vi "2_AdvancedDemo_MHHisto.vi"() -> ()   [LabVIEW 2010]
uses:
  Types/MH_UIThread_Cmds.ctl
  _lib/PQ/MultiHarp/MH_InitInfo.ctl
  Types/MH_UIThread_Data.ctl
  Types/MH_InputChannel.ctl
  _lib/PQ/MultiHarp/MH_RefSource.ctl
  _lib/PQ/MultiHarp/mhlib_x86_x64_UIThread.llb/MH_DllPath_global.vi
  <vilib>/Utility/error.llb/DialogType.ctl
  _lib/PQ/MultiHarp/MH_LibVersion_global.vi
  _lib/PQ/MultiHarp/MH_MeasMode.ctl
  Types/MH_SetInpChanData.ctl
  Types/MH_SetInpChanCmds.ctl
panel:
  in  "Settings":bool=TRUE
  in  "Run continuously":bool=TRUE caption="Conti."
  in  "Start":bool
  in  "Scale":bool
  out "CountRates":i32[](graph)
  in  "AllChannels":T1={"Enable"=TRUE, "Offset"=0, "Level"=-100, "Edge"=0, "DeadTime"=1000, "UseDeadTime"=FALSE, "SetEnableAllChan"=TRUE, "SetEdgeAllChan"=TRUE, "SetLevelAllChan"=TRUE, "SetOffsetAllChan"=TRUE, "SetUseDTAllChan"=TRUE, "SetDeadTAllChan"=TRUE} {"DeadTime" min=800 max=160000 step=1; "Edge" items=["falling", "rising"]; "Offset" min=-100000 max=100000 step=80; "Level" min=-1200 max=1200 step=1}
  in  "HistoLength":i32(ring)=6 caption="Num Bins" items=["1024", "2048", "4096", "8192", "16384", "32768", "65536"]
  in  "OvlLevel":u32=4294967295 caption="Ovl.Level" min=1 step=1
  in  "StopOvl.":bool=TRUE
  in  "AcqTime":i32=1000 caption="Acqu.           ms" min=1 max=360000 step=1
  in  "Binning":i32(ring) caption="Resol.            ps" items=["80", "160", "320", "640", "1280", "2560", "5120", "10240", "20480", "40960", "81920", "163840", "327680", "655360", "1310720", "2621440", "5242880", "10485760", "20971520", "41943040", "83886080", "167772160", "335544320"]
  in  "HistoOffset":i32 caption="Offset            ns" min=0 max=100000000 step=1
  out "HistoGraph":T2(graph)={0.0, "Resolution"=0.08, "Histogram"=[]}
  in  "SyncDeadTime":i32=1000 caption="Dead T.   ps" min=800 max=160000 step=1
  in  "UseDeadTime":bool caption="Use DT."
  in  "SyncEdge":i32(ring) caption="Edge" items=["falling", "rising"]
  in  "SyncDivider":i32(ring) caption="Divider" items=["1", "2", "4", "8", "16"]
  in  "SyncOffset":i32 caption="Offset      ps" min=-100000 max=100000 step=80
  in  "SyncLevel":i32=-100 caption="Level      mV" min=-1200 max=1200 step=1
  in  "Channels":T3[](array[typedef])=[{"Name"="Inp.Chan 1", "Enable"=TRUE, "Edge"=0, "Level"=-100, "Offset"=0, "UseDeadTime"=FALSE, "DeadTime"=1000}, {"Name"="Inp.Chan 2", "Enable"=TRUE, "Edge"=0, "Level"=-100, "Offset"=0, "UseDeadTime"=FALSE, "DeadTime"=1000}, {"Name"="Inp.Chan 3", "Enable"=TRUE, "Edge"=0, "Level"=-100, "Offset"=0, "UseDeadTime"=FALSE, "DeadTime"=1000}, {"Name"="Inp.Chan 4", "Enable"=TRUE, "Edge"=0, "Level"=-100, "Offset"=0, "UseDeadTime"=FALSE, "DeadTime"=1000}, {"Name"="Inp.Chan 5", "Enable"=TRUE, "Edge"=0, "Level"=-100, "Offset"=0, "UseDeadTime"=FALSE, "DeadTime"=1000}, {"Name"="Inp.Chan 6", "Enable"=TRUE, "Edge"=0, "Level"=-100, "Offset"=0, "UseDeadTime"=FALSE, "DeadTime"=1000}, {"Name"="Inp.Chan 7", "Enable"=TRUE, "Edge"=0, "Level"=-100, "Offset"=0, "UseDeadTime"=FALSE, "DeadTime"=1000}, {"Name"="Inp.Chan 8", "Enable"=TRUE, "Edge"=0, "Level"=-100, "Offset"=0, "UseDeadTime"=FALSE, "DeadTime"=1000}, {"Name"="Inp.Chan 9", "Enable"=TRUE, "Edge"=0, "Level"=-100, "Offset"=0, "UseDeadTime"=FALSE, "DeadTime"=1000}, {"Name"="Inp.Chan 10", "Enable"=TRUE, "Edge"=0, "Level"=-100, "Offset"=0, "UseDeadTime"=FALSE, "DeadTime"=1000}, {"Name"="Inp.Chan 11", "Enable"=TRUE, "Edge"=0, "Level"=-100, "Offset"=0, "UseDeadTime"=FALSE, "DeadTime"=1000}, {"Name"="Inp.Chan 12", "Enable"=TRUE, "Edge"=0, "Level"=-100, "Offset"=0, "UseDeadTime"=FALSE, "DeadTime"=1000}, {"Name"="Inp.Chan 13", "Enable"=TRUE, "Edge"=0, "Level"=-100, "Offset"=0, "UseDeadTime"=FALSE, "DeadTime"=1000}, {"Name"="Inp.Chan 14", "Enable"=TRUE, "Edge"=0, "Level"=-100, "Offset"=0, "UseDeadTime"=FALSE, "DeadTime"=1000}, {"Name"="Inp.Chan 15", "Enable"=TRUE, "Edge"=0, "Level"=-100, "Offset"=0, "UseDeadTime"=FALSE, "DeadTime"=1000}, {"Name"="Inp.Chan 16", "Enable"=TRUE, "Edge"=0, "Level"=-100, "Offset"=0, "UseDeadTime"=FALSE, "DeadTime"=1000}] {"DeadTime" min=800 max=160000 step=1; "Edge" items=["falling", "rising"]; "Offset" min=-100000 max=100000 step=80; "Level" min=-1200 max=1200 step=1}
  out "SyncRate":string="Sync Rate: 4999950 cps\n"
  out "OverFlow":bool caption="Overflow:"
  out "Status":string="Readout Rate: 8.6 Hz\t\tTotal Counts:\t\tCh. 1: 0 cnts.\t\tCh. 2: 1962112 cnts.\t\tCh. 3: 0 cnts.\t\tCh. 4: 1962112 cnts.\t\tCh. 5: 0 cnts.\t\tCh. 6: 1962112 cnts.\t\tCh. 7: 0 cnts.\t\tCh. 8: 1962112 cnts.\t\tCh. 9: 1962113 cnts.\t\tCh.10: 0 cnts.\t\tCh.11: 1962113 cnts.\t\tCh.12: 0 cnts.\t\tCh.13: 1962113 cnts.\t\tCh.14: 0 cnts.\t\tCh.15: 1962113 cnts.\t\tCh.16: 1962113 cnts.\t\t"
  # "Acquisition"
  # "All Channels"
  # "Sync"
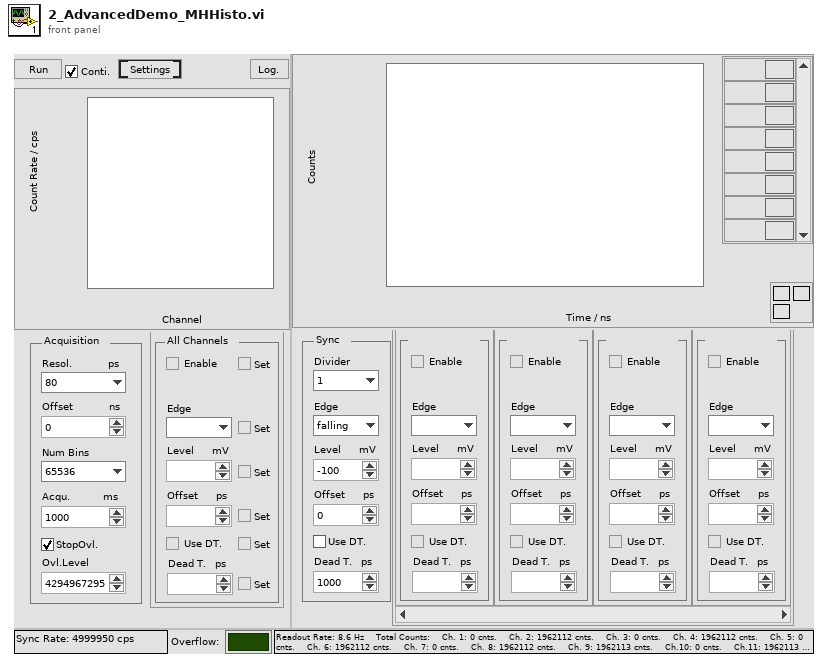
[diagram p1: front panel]
types:
  T1 = cluster{"Enable":bool, "Offset":i32, "Level":i32, "Edge":i32, "DeadTime":i32, "UseDeadTime":bool, "SetEnableAllChan":bool, "SetEdgeAllChan":bool, "SetLevelAllChan":bool, "SetOffsetAllChan":bool, "SetUseDTAllChan":bool, "SetDeadTAllChan":bool}
  T2 = cluster{dbl, "Resolution":dbl, "Histogram":u32[][]}
  T3 = typedef "MH_InputChannel.ctl" = cluster{"Name":string, "Enable":bool, "Edge":i32, "Level":i32, "Offset":i32, "UseDeadTime":bool, "DeadTime":i32}
  T4 = typedef "MH_UIThread_Data.ctl" = cluster{"Init Info":T5, "DevIdx":i32, "SyncDivider":i32, "SyncOffset":i32, "SyncLevel":i32, "Channels":T3[], "CurrentChannels":i32[], "AcqTime":i32, "Binning":i32, "HistoOffset":i32, "HistoLen":i32, "StopOvl.":bool, "OvlLevel":u32, "SyncEdge":i32, "StartMeas":bool, "HistoLength":i32, "Resolution":dbl, "Run cont.":bool, "Status":string, "SyncRate":i32, "BitShift":i32, "HistoAcqTime":dbl, "SyncRateStart":i32, "UseDeadTime":bool, "SyncDeadTime":i32, "SetInpChan":T6[]}
  T5 = typedef "MH_InitInfo.ctl" = cluster{"Library Version":string, "Serial No.":string, "Model":string, "Partnum":string, "Version":string, "features":i32, "nchannels":i32, "Base Resolution":dbl, "Bin Steps":i32}
  T6 = typedef "MH_SetInpChanData.ctl" = cluster{"Channel":i32, "Cmds":T7[], "Changed":cluster{"Name":bool, "Enable":bool, "Edge":bool, "Level":bool, "Offset":bool, "UseDeadTime":bool, "DeadTime":bool}}
  T7 = typedef "MH_SetInpChanCmds.ctl" = enum16{"SetInpChanEnable", "SetInpChanOffset", "SetInpChanDeadTime", "SetInpChanTrg"}
  T8 = typedef "MH_UIThread_Cmds.ctl" = enum16{"Idle", "Init", "SetInpChan", "SetSyncDivider", "SetSyncTrg", "SetSyncOffset", "SetSyncDeadTime", "SetBinning", "SetHistoOffset", "SetHistoLen", "SetStopOvl", "SetBitShift", "SetHistoAcqTime", "GetRates", "GetAllRates", "StartMeas", "StopMeas", "AbortMeas", "GetResolution", "GetHistos", "GetAllHistos", "ReadFiFo", "WriteStatus", "Resize", "EnableControls", "DisableControls", "Error", "Exit"}
  T9 = enum8{"Enabled", "Disabled", "Disabled and Grayed Out"}
  T10 = cluster{"[0]":bool, "[1]":bool, "[2]":bool, "[3]":bool, "[4]":bool, "[5]":bool}
  T11 = typedef "MH_MeasMode.ctl" = i32
  T12 = typedef "MH_RefSource.ctl" = enum16{"INTERNAL", "EXTERNAL_10MHZ", "WR_MASTER_GENERIC", "WR_SLAVE_GENERIC", "WR_GRANDM_GENERIC", "EXTN_GPS_PPS", "EXTN_GPS_PPS_UART", "WR_MASTER_MHARP", "WR_SLAVE_MHARP", "WR_GRANDM_MHARP"}
  T13 = cluster{dbl, "Resolution":dbl, "Histograms":u32[][]}
  T14 = typedef "DialogType.ctl" = u16
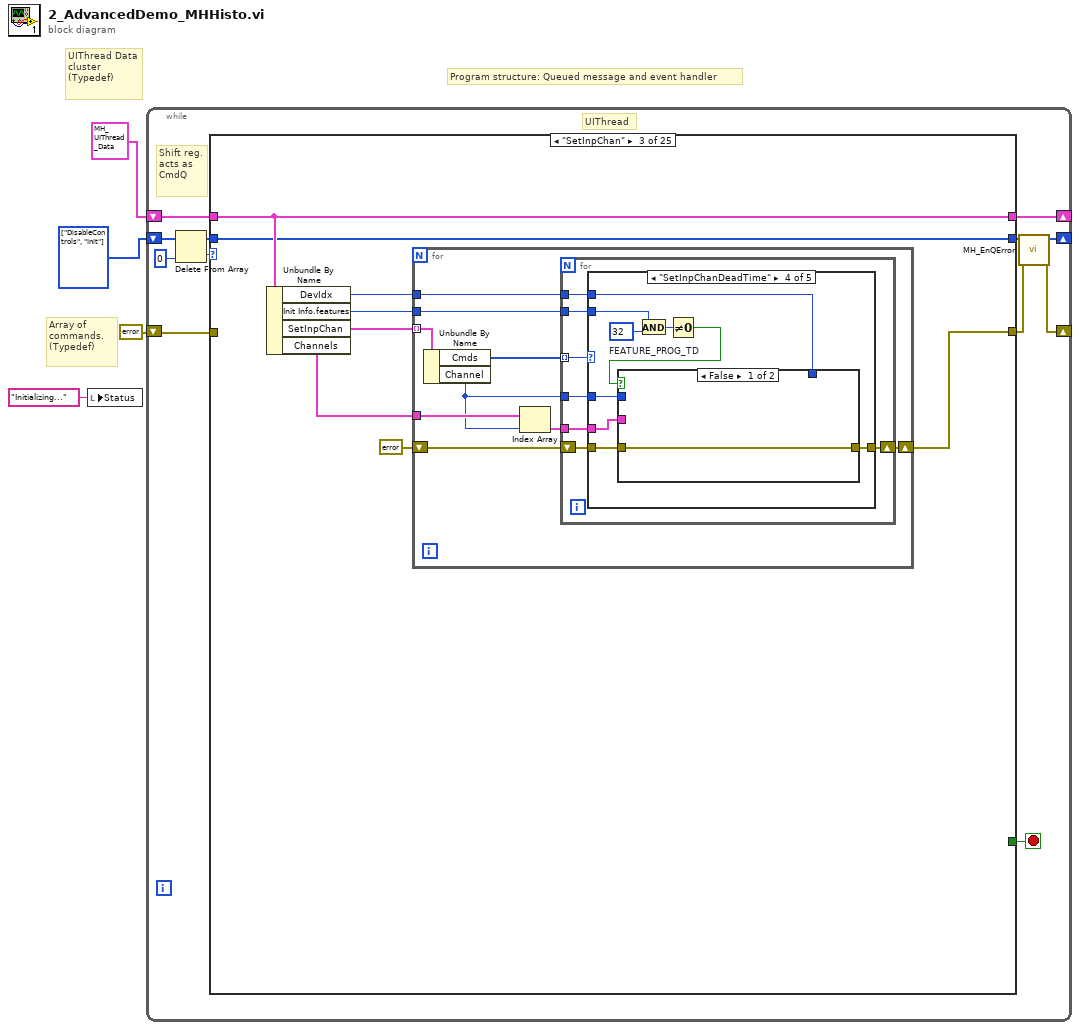
[diagram p0: block diagram]
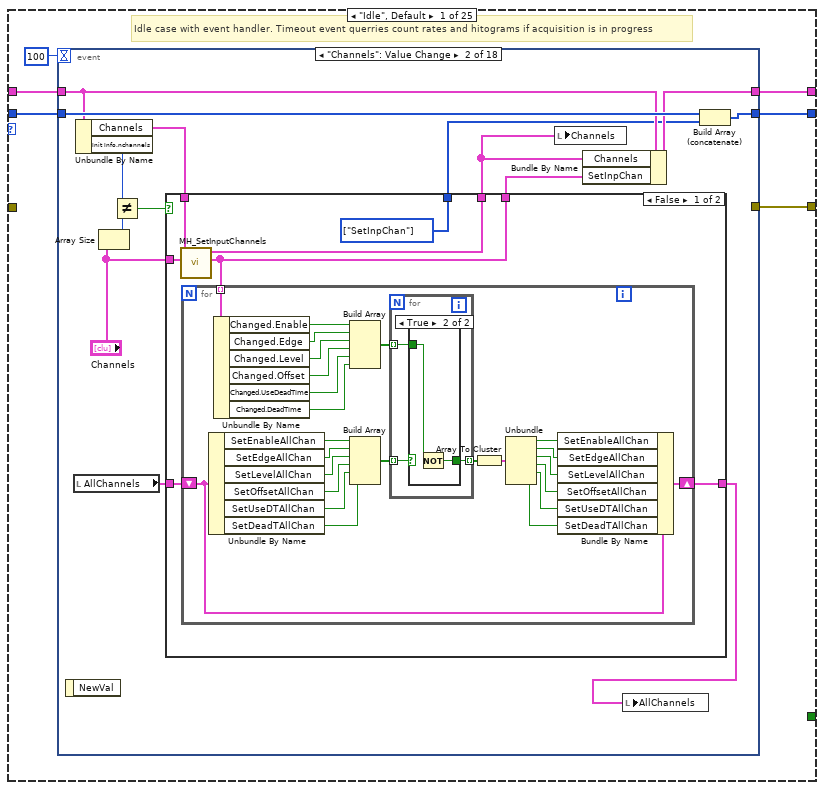
[diagram p2: hidden frame]
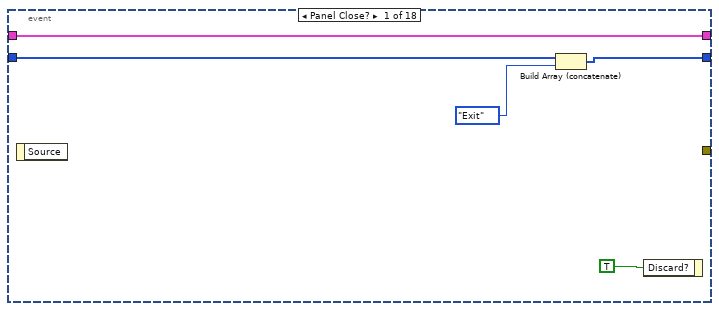
[diagram p3: hidden frame]
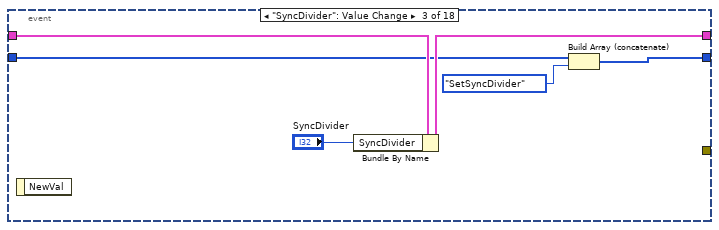
[diagram p6: hidden frame]
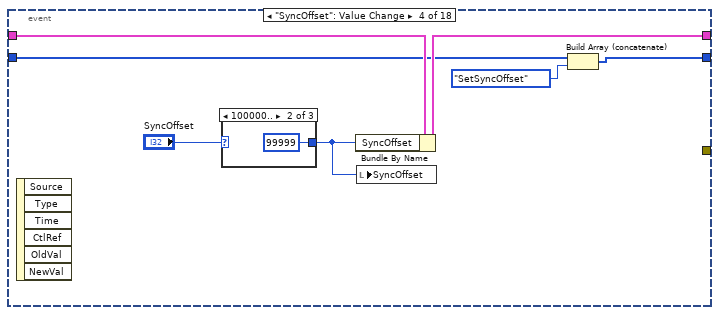
[diagram p7: hidden frame]
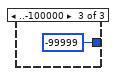
[diagram p9: hidden frame]
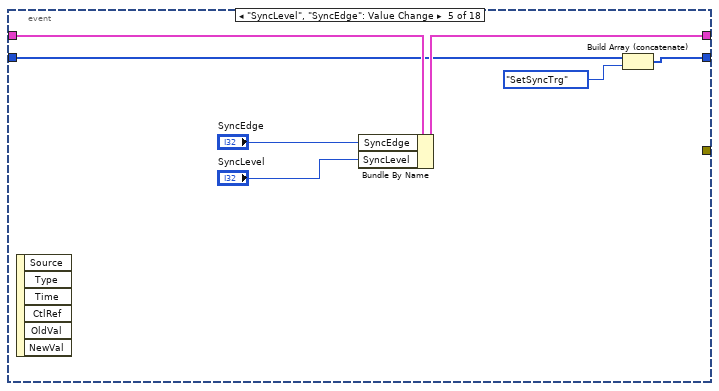
[diagram p10: hidden frame]
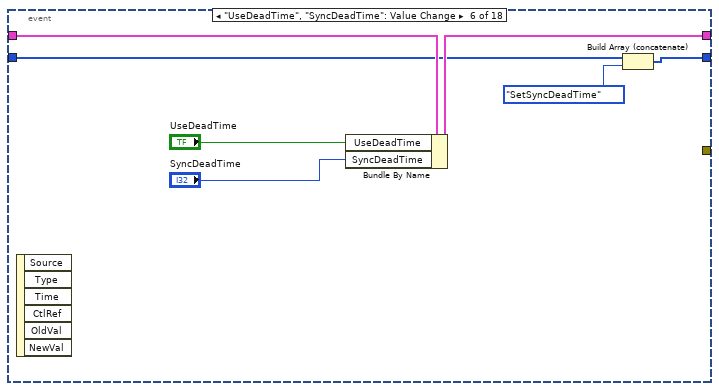
[diagram p11: hidden frame]
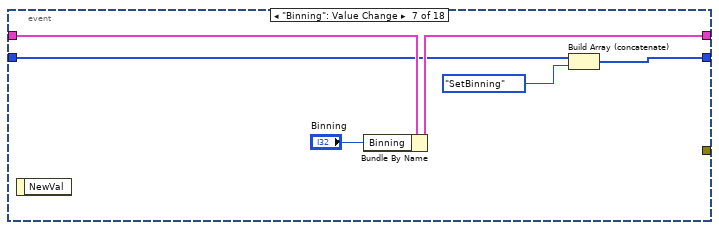
[diagram p12: hidden frame]
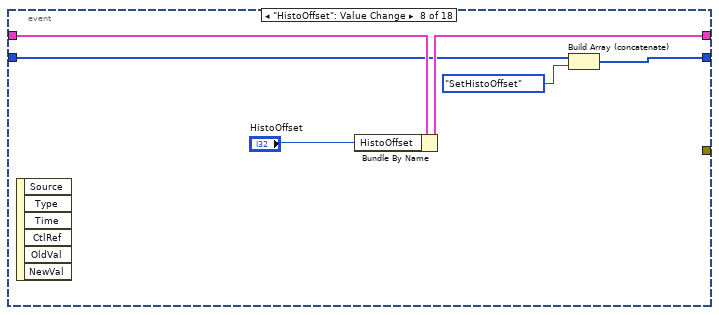
[diagram p13: hidden frame]
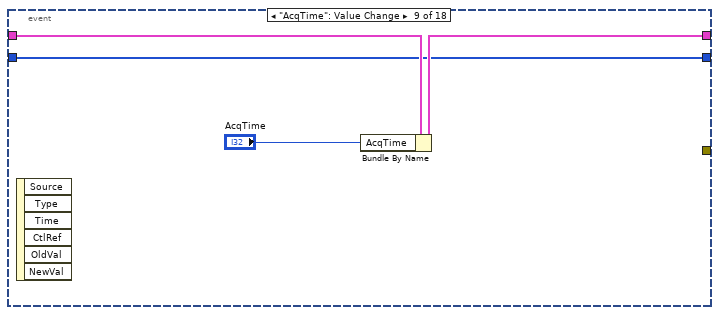
[diagram p14: hidden frame]
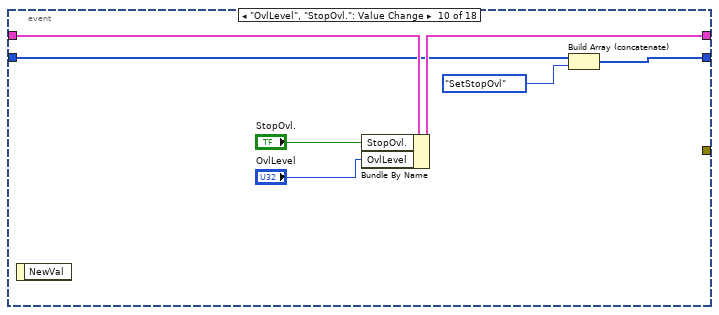
[diagram p15: hidden frame]
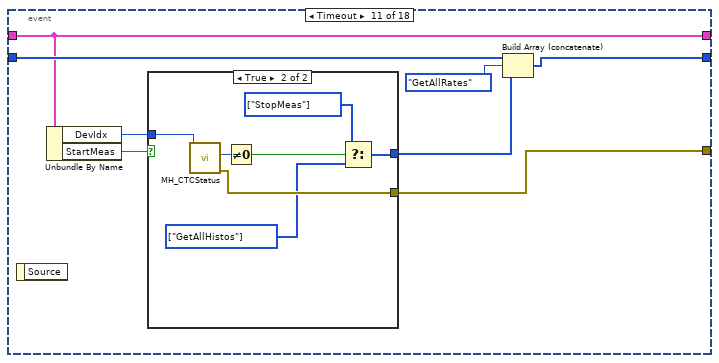
[diagram p16: hidden frame]
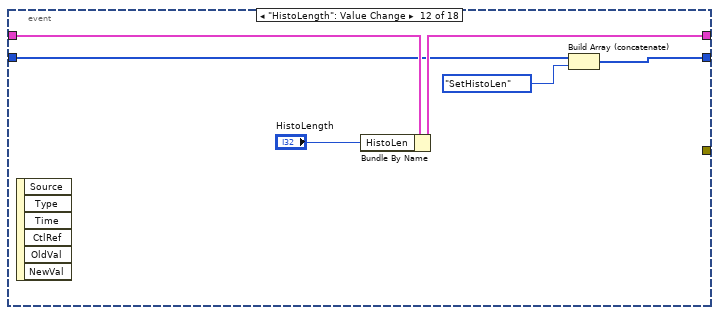
[diagram p18: hidden frame]
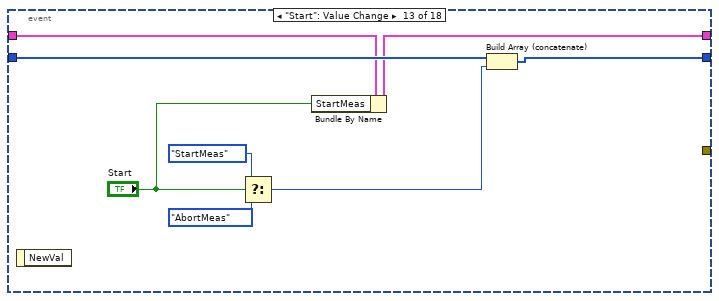
[diagram p19: hidden frame]
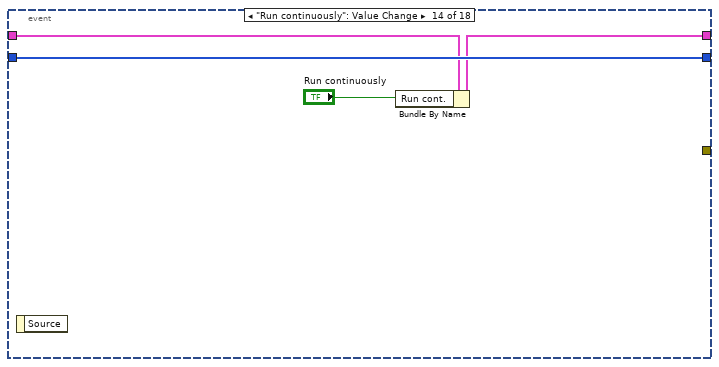
[diagram p20: hidden frame]
diagram:
  w3 = T8[] [enum."DisableControls", enum."Init"] items=["Idle", "Init", "SetInpChan", "SetSyncDivider", "SetSyncTrg", "SetSyncOffset", "SetSyncDeadTime", "SetBinning", "SetHistoOffset", "SetHistoLen", "SetStopOvl", "SetBitShift", "SetHistoAcqTime", "GetRates", "GetAllRates", "StartMeas", "StopMeas", "AbortMeas", "GetResolution", "GetHistos", "GetAllHistos", "ReadFiFo", "WriteStatus", "Resize", "EnableControls", "DisableControls", "Error", "Exit"]
  # "Array of commands.\n(Typedef)"
  # "Program structure: Queued message and event handler"
  # "UIThread Data cluster\n(Typedef)"
  n1 = local write "Status"("Initializing..." ("Status")) -> ()
  n2 = while {
    shift-right: [w5] -> _
    shift-left: w3 -> [w12]
    shift-right: [w15] -> _
    shift-left: T4 {"Init Info"={"Library Version"="", "Serial No."="", "Model"="", "Partnum"="", "Version"="", "features"=0, "nchannels"=0, "Base Resolution"=0.0, "Bin Steps"=0}, "DevIdx"=0, "SyncDivider"=1, "SyncOffset"=0, "SyncLevel"=50, "Channels"=[], "CurrentChannels"=[], "AcqTime"=1, "Binning"=1, "HistoOffset"=1, "HistoLen"=1024, "StopOvl."=FALSE, "OvlLevel"=1024, "SyncEdge"=10, "StartMeas"=FALSE, "HistoLength"=0, "Resolution"=0.0, "Run cont."=FALSE, "Status"="", "SyncRate"=0, "BitShift"=0, "HistoAcqTime"=0.0, "SyncRateStart"=0, "UseDeadTime"=FALSE, "SyncDeadTime"=800, "SetInpChan"=[]} -> [w14]
    shift-right: [w7] -> _
    shift-left: errorcluster {"status"=FALSE, "code"=0, "source"=""} ("error IO") -> [w13]
    stop <- w16 stop-if-true
    # "Shift reg.\nacts as\nCmdQ"
    # "UIThread"
    n3 = Delete From Array(array=w12, index=0) -> (deleted portion=w10:T8, array with subset deleted=w9:T8[])  [unwired: 1 in]
    n4 = case shown="\"SetInpChan\"" w10 {
      tunnel: [w22 w304 w323 w385 w394 w406 w412 w419 w427 w435 w440 w451 w462 w477 w485 w499 w513 w538 w570 w594 w607 w614 w626 w632 w636] -> w6
      tunnel: [_ _ _ _ _ _ _ _ _ _ _ _ _ _ _ _ _ _ _ _ _ _ _ _ TRUE] -> w16
      tunnel: [w21 w284 w324 w387 w395 w407 w416 w423 w428 w430 w441 w450 w461 w483 w488 w502 w509 w537 w569 w593 w595 w613 w625 w633 w639] -> w15
      tunnel: w14 -> [w20 w289 w324 w387 w395 w407 w416 w423 w428 w431 w441 w450 w461 w483 w489 w503 w510 w537 w569 w593 w595 w613 w625 w633 w639]
      tunnel: [w17 w307 w321 w383 w393 w405 w415 w422 w426 w434 w439 w444 w460 w482 w491 w505 w511 w535 w565 _ _ _ _ _ w637] -> w8
      tunnel: w13 -> [_ _ _ _ _ _ _ _ _ _ _ _ _ _ _ _ _ _ _ _ _ _ _ w634 _]
      tunnel: w9 -> [w19 w306 w323 w385 w394 w406 w412 w418 w427 w435 w440 w451 w462 w478 w486 w500 w513 w538 w570 w594 w607 w614 w626 _ w636]
      frame "Idle", Default {
        # "Idle case with event handler. Timeout event querries count rates and hitograms if acquisition is in progress"
        n5 = event shown="[1] \"Channels\": Value Change" {
          selector: _ -> [_ _ _ _ _ _ _ _ _ _ _ _ _ _ _ _ _ _]
          dyn-events: _ -> [_ _ _ _ _ _ _ _ _ _ _ _ _ _ _ _ _ _]
          timeout: 100 -> [_ _ _ _ _ _ _ _ _ _ _ _ _ _ _ _ _ _]
          tunnel: [w23 w40 w82 w90 w99 w107 w113 w119 w124 w130 w140 w151 w159 w167 w173 w181 w191 w204] -> w22
          tunnel: [w26 w33 w86 w93 w103 w110 w116 w122 w126 w133 w139 w154 w157 w165 w172 w180 w194 w198] -> w21
          tunnel: w20 -> [w26 w35 w87 w94 w104 w111 w117 w123 w127 w134 w139 w155 w158 w166 w172 w180 w194 w199]
          tunnel: w19 -> [w25 w41 w84 w92 w101 w109 w115 w121 w124 w132 w142 w153 w161 w167 w173 w181 w192 w205]
          tunnel: [_ _ _ _ _ _ _ _ _ _ w135 _ _ _ _ _ _ _] -> w17
          event Panel Close? {
            n6 = event-data() -> ()  [unwired: 1 in, 1 out]
            n7 = Build Array (concatenate)(w25, MH_UIThread_Cmds."Exit") -> (w23:T8[])
            n8 = event-data("Discard?"=TRUE) -> ()  [unwired: 1 in, 1 out]
          }
          event "Channels": Value Change {
            n9 = event-data() -> ()  [unwired: 1 in, 1 out]
            n10 = local read "AllChannels"() -> (w29:T1)
            n11 = Unbundle By Name(w35) -> ("Channels"=w36:T3[], "Init Info.nchannels"=w39:i32)
            n12 = Array Size(array="Channels") -> (size(s)=w38:i32)
            n13 = Not Equal?(x=w39, y=w38) -> (x != y?=w37:bool)
            n14 = case shown="False" w37 {
              tunnel: "Channels" -> [w47 _]
              tunnel: [w46 w81] -> w34
              tunnel: w36 -> [w48 w81]
              tunnel: [w44 _] -> w32
              tunnel: [w45 _] -> w30
              tunnel: w29 -> [w43 w80]
              tunnel: [w42 w80] -> w28
              frame False {
                w45 = T8[] [enum."SetInpChan"] items=["Idle", "Init", "SetInpChan", "SetSyncDivider", "SetSyncTrg", "SetSyncOffset", "SetSyncDeadTime", "SetBinning", "SetHistoOffset", "SetHistoLen", "SetStopOvl", "SetBitShift", "SetHistoAcqTime", "GetRates", "GetAllRates", "StartMeas", "StopMeas", "AbortMeas", "GetResolution", "GetHistos", "GetAllHistos", "ReadFiFo", "WriteStatus", "Resize", "EnableControls", "DisableControls", "Error", "Exit"] ("array")
                n15 = call "MH_SetInputChannels.vi"("Channels new"=w47, "Channels old"=w48) -> ("SetInpChan"=w44:T6[], "Channels"=w46:T3[])  [unwired: 8 in]
                n16 = for {
                  tunnel: w44 -> [w73] mode=indexing
                  shift-right: [w55] -> w42
                  shift-left: w43 -> [w57]
                  n17 = Unbundle By Name(w57) -> ("SetEnableAllChan"=w66:bool, "SetEdgeAllChan"=w65:bool, "SetLevelAllChan"=w64:bool, "SetOffsetAllChan"=w63:bool, "SetUseDTAllChan"=w62:bool, "SetDeadTAllChan"=w61:bool)
                  n18 = Unbundle By Name(w73) -> ("Changed.Enable"=w72:bool, "Changed.Edge"=w71:bool, "Changed.Level"=w70:bool, "Changed.Offset"=w69:bool, "Changed.UseDeadTime"=w68:bool, "Changed.DeadTime"=w67:bool)
                  n19 = Build Array(w72, w71, w70, w69, w68, w67) -> (w59:bool[])
                  n20 = Build Array(w66, w65, w64, w63, w62, w61) -> (w60:bool[])
                  n21 = for {
                    tunnel: w60 -> [w76] mode=indexing
                    tunnel: w59 -> [w74] mode=indexing
                    tunnel: [w75] -> w58 mode=indexing
                    n22 = case shown="True" w76 {
                      selector: w76 -> [w77 _]
                      tunnel: [w77 w78] -> w75
                      tunnel: w74 -> [_ w79]
                      frame False {
                      }
                      frame True {
                        n23 = Not(x=w79) -> (.not. x?=w78:bool)
                      }
                    }
                  }
                  n24 = Array To Cluster(array=w58) -> (cluster=w56:T10)
                  n25 = Unbundle(w56) -> ("[0]"=w54:bool, "[1]"=w53:bool, "[2]"=w52:bool, "[3]"=w51:bool, "[4]"=w50:bool, "[5]"=w49:bool)
                  n26 = Bundle By Name(cluster=w57, "SetEnableAllChan"=w54, "SetEdgeAllChan"=w53, "SetLevelAllChan"=w52, "SetOffsetAllChan"=w51, "SetUseDTAllChan"=w50, "SetDeadTAllChan"=w49) -> (w55:T1)
                }
              }
              frame True {
              }
            }
            n27 = local write "Channels"(w34) -> ()
            n28 = Bundle By Name(cluster=w35, "Channels"=w34, "SetInpChan"=w32) -> (w33:T4)
            n29 = local write "AllChannels"(w28) -> ()
            n30 = Build Array (concatenate)(w41, w30) -> (w40:T8[])
          }
          event "SyncDivider": Value Change {
            n31 = event-data() -> ()  [unwired: 1 in, 1 out]
            n32 = Bundle By Name(cluster=w87, "SyncDivider"="SyncDivider") -> (w86:T4)
            n33 = Build Array (concatenate)(w84, MH_UIThread_Cmds."SetSyncDivider") -> (w82:T8[])
          }
          event "SyncOffset": Value Change {
            n34 = event-data() -> ()  [unwired: 1 in, 6 out]
            n35 = case shown="100000.." "SyncOffset" {
              selector: "SyncOffset" -> [w95 _ _]
              tunnel: [w95 99999 ("SyncOffset") -99999 ("SyncOffset")] -> w88
              frame Default {
              }
              frame 100000.. {
              }
              frame ..-100000 {
              }
            }
            n36 = Bundle By Name(cluster=w94, "SyncOffset"=w88) -> (w93:T4)
            n37 = local write "SyncOffset"(w88) -> ()
            n38 = Build Array (concatenate)(w92, MH_UIThread_Cmds."SetSyncOffset") -> (w90:T8[])
          }
          event "SyncLevel", "SyncEdge": Value Change {
            n39 = event-data() -> ()  [unwired: 1 in, 6 out]
            n40 = Bundle By Name(cluster=w104, "SyncEdge"="SyncEdge", "SyncLevel"="SyncLevel") -> (w103:T4)
            n41 = Build Array (concatenate)(w101, MH_UIThread_Cmds."SetSyncTrg") -> (w99:T8[])
          }
          event "UseDeadTime", "SyncDeadTime": Value Change {
            n42 = event-data() -> ()  [unwired: 1 in, 6 out]
            n43 = Bundle By Name(cluster=w111, "UseDeadTime"="UseDeadTime", "SyncDeadTime"="SyncDeadTime") -> (w110:T4)
            n44 = Build Array (concatenate)(w109, MH_UIThread_Cmds."SetSyncDeadTime") -> (w107:T8[])
          }
          event "Binning": Value Change {
            n45 = event-data() -> ()  [unwired: 1 in, 1 out]
            n46 = Bundle By Name(cluster=w117, "Binning"="Binning") -> (w116:T4)
            n47 = Build Array (concatenate)(w115, MH_UIThread_Cmds."SetBinning") -> (w113:T8[])
          }
          event "HistoOffset": Value Change {
            n48 = event-data() -> ()  [unwired: 1 in, 6 out]
            n49 = Bundle By Name(cluster=w123, "HistoOffset"="HistoOffset") -> (w122:T4)
            n50 = Build Array (concatenate)(w121, MH_UIThread_Cmds."SetHistoOffset") -> (w119:T8[])
          }
          event "AcqTime": Value Change {
            n51 = event-data() -> ()  [unwired: 1 in, 6 out]
            n52 = Bundle By Name(cluster=w127, "AcqTime"="AcqTime") -> (w126:T4)
          }
          event "OvlLevel", "StopOvl.": Value Change {
            n53 = event-data() -> ()  [unwired: 1 in, 1 out]
            n54 = Bundle By Name(cluster=w134, "StopOvl."="StopOvl.", "OvlLevel"="OvlLevel") -> (w133:T4)
            n55 = Build Array (concatenate)(w132, MH_UIThread_Cmds."SetStopOvl") -> (w130:T8[])
          }
          event Timeout {
            n56 = event-data() -> ()  [unwired: 1 in, 1 out]
            n57 = Unbundle By Name(w139) -> ("DevIdx"=w137:i32, "StartMeas"=w138:bool)
            n58 = case shown="True" w138 {
              tunnel: w137 -> [_ w149]
              tunnel: [_ w147] -> w136
              tunnel: [_ w145] -> w135
              frame False {
              }
              frame True {
                w143 = T8[] [enum."GetAllHistos"] items=["Idle", "Init", "SetInpChan", "SetSyncDivider", "SetSyncTrg", "SetSyncOffset", "SetSyncDeadTime", "SetBinning", "SetHistoOffset", "SetHistoLen", "SetStopOvl", "SetBitShift", "SetHistoAcqTime", "GetRates", "GetAllRates", "StartMeas", "StopMeas", "AbortMeas", "GetResolution", "GetHistos", "GetAllHistos", "ReadFiFo", "WriteStatus", "Resize", "EnableControls", "DisableControls", "Error", "Exit"]
                w146 = T8[] [enum."StopMeas"] items=["Idle", "Init", "SetInpChan", "SetSyncDivider", "SetSyncTrg", "SetSyncOffset", "SetSyncDeadTime", "SetBinning", "SetHistoOffset", "SetHistoLen", "SetStopOvl", "SetBitShift", "SetHistoAcqTime", "GetRates", "GetAllRates", "StartMeas", "StopMeas", "AbortMeas", "GetResolution", "GetHistos", "GetAllHistos", "ReadFiFo", "WriteStatus", "Resize", "EnableControls", "DisableControls", "Error", "Exit"]
                n59 = call "MH_CTCStatus.vi"("devidx"=w149) -> ("error out"=w145:errorcluster, "ctcstatus"=w148:i32)  [unwired: 8 in, 1 out]
                n60 = Not Equal To 0?(x=w148) -> (x != 0?=w144:bool)
                n61 = Select(t=w146, s=w144, f=w143) -> (s? t:f=w147:T8[])
              }
            }
            n62 = Build Array (concatenate)(w142, MH_UIThread_Cmds."GetAllRates", w136) -> (w140:T8[])
          }
          event "HistoLength": Value Change {
            n63 = event-data() -> ()  [unwired: 1 in, 6 out]
            n64 = Bundle By Name(cluster=w155, "HistoLen"="HistoLength") -> (w154:T4)
            n65 = Build Array (concatenate)(w153, MH_UIThread_Cmds."SetHistoLen") -> (w151:T8[])
          }
          event "Start": Value Change {
            n66 = event-data() -> ()  [unwired: 1 in, 1 out]
            n67 = Select(t=MH_UIThread_Cmds."StartMeas", s="Start", f=MH_UIThread_Cmds."AbortMeas") -> (s? t:f=w160:T8)
            n68 = Bundle By Name(cluster=w158, "StartMeas"="Start") -> (w157:T4)
            n69 = Build Array (concatenate)(w161, w160) -> (w159:T8[])
          }
          event "Run continuously": Value Change {
            n70 = event-data() -> ()  [unwired: 1 in, 1 out]
            n71 = Bundle By Name(cluster=w166, "Run cont."="Run continuously") -> (w165:T4)
          }
          event "Scale": Value Change {
            n72 = event-data() -> ()  [unwired: 1 in, 1 out]
            n73 = Select(t=u8 0 ("Y Scale.Mapping Mode"), s="Scale", f=u8 1 ("Y Scale.Mapping Mode")) -> (s? t:f=w168:u8)
            n74 = property on="HistoGraph" class="WFGraph (strict)"("YScale.Mapping Mode"=w168) -> ()  [unwired: 2 in, 2 out]
          }
          event "Settings": Value Change {
            n75 = event-data() -> ()  [unwired: 1 in, 1 out]
            n76 = property on="Splitter" class="Splitter"() -> ("Position"=w179:i32)  [unwired: 2 in, 2 out]
            n77 = Select(t=300 ("PosT"), s="Settings", f=0 ("PosF")) -> (s? t:f=w176:i32)
            n78 = Subtract(x=w179, y=w176) -> (x-y=w175:i32)
            n79 = while {
              shift-right: [w190] -> _
              shift-left: w175 -> [w183]
              i -> [w189]
              stop <- w186 stop-if-true
              n80 = property on="Splitter 4" class="Splitter"("Position"=w183) -> (error out=w182:errorcluster)  [unwired: 2 in, 1 out]
              n81 = Greater Or Equal?(x=w189, y=10) -> (x >= y?=w187:bool)
              n82 = Decrement(x=w183) -> (x-1=w190:i32)
              n83 = Unbundle(w182) -> ("status"=w185:bool)  [unwired: 2 out]
              n84 = Not(x=w185) -> (.not. x?=w184:bool)
              n85 = Or(x=w184, y=w187) -> (x .or. y?=w186:bool)
            }
          }
          event Panel Resize {
            n86 = event-data() -> ()  [unwired: 1 in, 1 out]
            n87 = Build Array (concatenate)(w192, MH_UIThread_Cmds."Resize") -> (w191:T8[])
          }
          event "AllChannels": Value Change {
            w196 = T8[] [enum."SetInpChan"] items=["Idle", "Init", "SetInpChan", "SetSyncDivider", "SetSyncTrg", "SetSyncOffset", "SetSyncDeadTime", "SetBinning", "SetHistoOffset", "SetHistoLen", "SetStopOvl", "SetBitShift", "SetHistoAcqTime", "GetRates", "GetAllRates", "StartMeas", "StopMeas", "AbortMeas", "GetResolution", "GetHistos", "GetAllHistos", "ReadFiFo", "WriteStatus", "Resize", "EnableControls", "DisableControls", "Error", "Exit"] ("array")
            n88 = event-data() -> ()  [unwired: 1 in, 1 out]
            n89 = local read "Channels"() -> (w203:T3[])
            n90 = for {
              tunnel: w203 -> [w208] mode=indexing
              tunnel: "AllChannels" -> [w207]
              tunnel: [w206] -> w201 mode=indexing
              n91 = Unbundle By Name(w207) -> ("SetEnableAllChan"=w209:bool, "SetEdgeAllChan"=w210:bool, "SetLevelAllChan"=w211:bool, "SetOffsetAllChan"=w212:bool, "SetUseDTAllChan"=w213:bool, "SetDeadTAllChan"=w214:bool)
              n92 = Build Array(w209, w210, w211, w212, w213, w214) -> (w215:bool[])
              n93 = for {
                tunnel: w215 -> [w220] mode=indexing
                shift-right: [w217] -> w206
                shift-left: w208 -> [w218]
                tunnel: w207 -> [w216]
                i -> [w219]
                n94 = case shown="True" w220 {
                  tunnel: w219 -> [_ w225]
                  tunnel: w216 -> [_ w224]
                  tunnel: w218 -> [w221 w223]
                  tunnel: [w221 w222] -> w217
                  frame False {
                  }
                  frame True {
                    n95 = case shown="Default" w225 {
                      tunnel: w224 -> [w229 w233 w237 w242 w249 w253 _]
                      tunnel: w223 -> [w228 w232 w236 w241 w248 w252 w254]
                      tunnel: [w226 w230 w234 w240 w246 w250 w254] -> w222
                      frame 0 {
                        n96 = Unbundle By Name(w229) -> ("Enable"=w227:bool)
                        n97 = Bundle By Name(cluster=w228, "Enable"=w227) -> (w226:T3)
                      }
                      frame 1 {
                        n98 = Unbundle By Name(w233) -> ("Edge"=w231:i32)
                        n99 = Bundle By Name(cluster=w232, "Edge"=w231) -> (w230:T3)
                      }
                      frame 2 {
                        n100 = Unbundle By Name(w237) -> ("Level"=w235:i32)
                        n101 = Bundle By Name(cluster=w236, "Level"=w235) -> (w234:T3)
                      }
                      frame 3 {
                        n102 = Unbundle By Name(w242) -> ("Offset"=w239:i32)
                        n103 = case shown="100000.." w239 {
                          selector: w239 -> [w243 _ _]
                          tunnel: [w243 99999 ("SyncOffset") -99999 ("SyncOffset")] -> w238
                          frame Default {
                          }
                          frame 100000.. {
                          }
                          frame ..-100000 {
                          }
                        }
                        n104 = Bundle By Name(cluster=w241, "Offset"=w238) -> (w240:T3)
                      }
                      frame 4 {
                        n105 = Unbundle By Name(w249) -> ("UseDeadTime"=w247:bool)
                        n106 = Bundle By Name(cluster=w248, "UseDeadTime"=w247) -> (w246:T3)
                      }
                      frame 5 {
                        n107 = Unbundle By Name(w253) -> ("DeadTime"=w251:i32)
                        n108 = Bundle By Name(cluster=w252, "DeadTime"=w251) -> (w250:T3)
                      }
                      frame Default {
                      }
                    }
                  }
                }
              }
            }
            n109 = Build Array (concatenate)(w205, w196) -> (w204:T8[])
            n110 = Unbundle By Name(w199) -> ("Channels"=w200:T3[])
            n111 = call "MH_SetInputChannels.vi"("Channels new"=w201, "Channels old"=w200) -> ("SetInpChan"=w197:T6[], "Channels"=w195:T3[])  [unwired: 8 in]
            n112 = local write "Channels"(w195) -> ()
            n113 = Bundle By Name(cluster=w199, "Channels"=w195, "SetInpChan"=w197) -> (w198:T4)
          }
        }
      }
      frame "Init" {
        w264 = 1000 ("SyncDeadTime")
        w265 = FALSE ("UseDeadTime")
        w267 = T11 0 items=["HIST"=0, "T2"=2, "T3"=3]  # Mode
        w277 = MH_RefSource."INTERNAL"  # refsource
        w291 = TRUE ("Run cont.")
        w293 = FALSE ("StartMeas")
        w294 = u32 4294967295 ("OvlLevel")
        w295 = TRUE ("StopOvl.")
        w296 = 6 ("HistoLen")
        w297 = 1000 ("AcqTime")
        w298 = 0 ("HistoOffset")
        w299 = 0 ("Binning")
        w300 = -100 ("SyncLevel")
        w301 = 0 ("SyncZeroX")
        w302 = 0 ("SyncOffset")
        w303 = 0 ("SyncDivider")
        w305 = T8[] [enum."SetSyncDivider", enum."SetSyncOffset", enum."SetSyncTrg", enum."SetSyncDeadTime", enum."SetInpChan", enum."SetBinning", enum."SetHistoOffset", enum."SetHistoLen", enum."SetStopOvl", enum."Resize", enum."EnableControls", enum."WriteStatus"] items=["Idle", "Init", "SetInpChan", "SetSyncDivider", "SetSyncTrg", "SetSyncOffset", "SetSyncDeadTime", "SetBinning", "SetHistoOffset", "SetHistoLen", "SetStopOvl", "SetBitShift", "SetHistoAcqTime", "GetRates", "GetAllRates", "StartMeas", "StopMeas", "AbortMeas", "GetResolution", "GetHistos", "GetAllHistos", "ReadFiFo", "WriteStatus", "Resize", "EnableControls", "DisableControls", "Error", "Exit"]
        # "Init HW"
        # "Set path to mhlib.dll"
        # "Init all FP controls and corresponding copy in UIThread Data cluster"
        # "EnQ list of commands"
        # "Array with Inp.Chan."
        # "Initialization: 1. Init HW -> get # of channels -> make array for Inp.Channels\n2. Init all FP controls and corresponding fields in UIThread Data cluster\n3. EnQ list of commands for further initialization"
        n114 = disable-structure shown="TARGET_TYPE==Windows, Default" {
          disable-tunnel: ["MHLib64" ("name or relative path") "MHLib" ("name or relative path")] -> w266
          frame condition #0 (active) {
          }
          frame condition #1 {
          }
        }
        n115 = call <vilib>:"Error Cluster From Error Code.vi"("is warning? (False)"=FALSE, "show call chain? (False)"=TRUE, "error message (\"\")"="DLL not found!" ("error message (\"\")"), "error code (0)"=5000) -> ("error out"=w278:errorcluster)  [unwired: 5 in]
        n116 = call "GetDLLPath.vi"("DllName_32bit"="MHLib" ("name or relative path"), "DllName_64bit"=w266) -> ("file exists?"=w280:bool, "DLLPath"=w281:path)  [unwired: 8 in]
        n117 = global write "MH_DllPath_global.vi" "DllPath"(w281) -> ()
        n118 = Build Array (concatenate)(w306, w305) -> (w304:T8[])
        n119 = Select(t=errorcluster {"status"=FALSE, "code"=0, "source"=""} ("error IO"), s=w280, f=w278) -> (s? t:f=w285:errorcluster)
        n120 = property on="AllChannels" class="Clust (strict)"("Val(Sgnl)"=T1 {"Enable"=TRUE, "Offset"=0, "Level"=-100, "Edge"=0, "DeadTime"=1000, "UseDeadTime"=FALSE, "SetEnableAllChan"=TRUE, "SetEdgeAllChan"=TRUE, "SetLevelAllChan"=TRUE, "SetOffsetAllChan"=TRUE, "SetUseDTAllChan"=TRUE, "SetDeadTAllChan"=TRUE} ("AllChannels")) -> ()  [unwired: 2 in, 2 out]
        n121 = property on="HistoGraph" class="WFGraph (strict)"("LegPlotMin"=u32 8 ("Legend:Plot Minimum")) -> ()  [unwired: 2 in, 2 out]
        n122 = property on="Settings" class="Bool (strict)"("Val(Sgnl)"=TRUE ("Value (Signaling)")) -> ()  [unwired: 2 in, 2 out]
        n123 = global read "MH_LibVersion_global.vi" "Library Version"() -> (w276:string)
        n124 = property on="Scale" class="Bool (strict)"("Val(Sgnl)"=FALSE ("Value (Signaling)")) -> ()  [unwired: 2 in, 2 out]
        n125 = call "InitMH_UIThread.vi"("error in (no error)"=w285, "Mode"=w267, "refsource"=w277, "Library Version"=w276) -> ("error out"=w307:errorcluster, "Init Info"=w309:T5, "DevIdx"=w308:i32)  [unwired: 5 in]
        n126 = local write "SyncDivider"(w303) -> ()
        n127 = local write "SyncOffset"(w302) -> ()
        n128 = local write "SyncEdge"(w301) -> ()
        n129 = local write "SyncLevel"(w300) -> ()
        n130 = local write "UseDeadTime"(w265) -> ()
        n131 = local write "SyncDeadTime"(w264) -> ()
        n132 = local write "Binning"(w299) -> ()
        n133 = local write "HistoOffset"(w298) -> ()
        n134 = local write "AcqTime"(w297) -> ()
        n135 = local write "HistoLength"(w296) -> ()
        n136 = local write "StopOvl."(w295) -> ()
        n137 = local write "OvlLevel"(w294) -> ()
        n138 = local write "Start"(w293) -> ()
        n139 = local write "Run continuously"(w291) -> ()
        n140 = Bundle By Name(cluster=w289, "DevIdx"=w308, "Init Info"=w309, "Status"="Initialized!") -> (w288:T4)
        n141 = Unbundle By Name(w288) -> ("Init Info.Bin Steps"=w287:i32, "Init Info.Base Resolution"=w270:dbl, "Init Info.nchannels"=w262:i32)
        n142 = Initialize Array(u32 0, w262, 1024 ("dimension size")) -> (w269:u32[][])
        n143 = call "MH_InitChannels.vi"("nchannels"=w262) -> ("SetInpChan"=w260:T6[], "Channels"=w261:T3[])  [unwired: 9 in]
        n144 = Divide(x=w270, y=1000.0) -> (x/y=w271:dbl)
        n145 = call "MH_CalcBinningValues.vi"("Bin Steps"=w287) -> ("BinningValues"=w292:cluster{"String":string, "Value":i32}[])  [unwired: 10 in]
        n146 = Bundle(0.0, w271, w269) -> (w263:cluster{dbl, dbl, u32[][]})  [unwired: 1 in]
        n147 = for {
          N: w262 -> [_]
          tunnel: w263 -> [w312]
          i -> [w314]
          n148 = Increment(x=w314) -> (x+1=w313:i32)
          n149 = Format Into String(format string="Ch.%d", w313) -> (resulting string=w315:string)  [unwired: 2 in, 1 out]
          n150 = property on="HistoGraph" class="WFGraph (strict)"("Value"=w312, "Active Plot"=w314, "Plot.Plot Name"=w315) -> ()  [unwired: 2 in, 2 out]
        }
        n151 = property on="Binning" class="Ring (strict)"("StringsAndValues[]"=w292) -> ()  [unwired: 2 in, 2 out]
        n152 = local write "Channels"(w261) -> ()
        n153 = Bundle By Name(cluster=w288, "Channels"=w261, "SetInpChan"=w260, "SyncDivider"=w303, "SyncOffset"=w302, "SyncEdge"=w301, "SyncLevel"=w300, "UseDeadTime"=w265, "SyncDeadTime"=w264, "Binning"=w299, "HistoOffset"=w298, "AcqTime"=w297, "HistoLen"=w296, "StopOvl."=w295, "OvlLevel"=w294, "StartMeas"=w293, "Run cont."=w291) -> (w284:T4)
      }
      frame "SetInpChan" {
        n154 = Unbundle By Name(w324) -> ("DevIdx"=w319:i32, "Init Info.features"=w317:i32, "SetInpChan"=w322:T6[], "Channels"=w318:T3[])
        n155 = for {
          tunnel: w318 -> [w329]
          tunnel: w322 -> [w333] mode=indexing
          shift-right: [w331] -> w321
          shift-left: errorcluster {"status"=FALSE, "code"=0, "source"=""} ("error out") -> [w330]
          tunnel: w319 -> [w327]
          tunnel: w317 -> [w325]
          n156 = Unbundle By Name(w333) -> ("Cmds"=w332:T7[], "Channel"=w326:i32)
          n157 = Index Array(array=w329, index=w326) -> (element=w328:T3)
          n158 = for {
            tunnel: w332 -> [w340] mode=indexing
            tunnel: w326 -> [w339]
            shift-right: [w338] -> w331
            shift-left: w330 -> [w337]
            tunnel: w328 -> [w336]
            tunnel: w327 -> [w335]
            tunnel: w325 -> [w334]
            n159 = case shown="\"SetInpChanDeadTime\"" w340 {
              tunnel: w339 -> [_ w346 w353 w358 w374]
              tunnel: [w341 w345 w352 w362 w379] -> w338
              tunnel: w337 -> [w341 w344 w351 w361 w378]
              tunnel: w336 -> [_ w343 w350 w360 w377]
              tunnel: w335 -> [_ w342 w349 w359 w376]
              tunnel: w334 -> [_ _ _ w355 _]
              frame Default {
              }
              frame "SetInpChanEnable" {
                n160 = Unbundle By Name(w343) -> ("Enable"=w347:bool)
                n161 = call "MH_SetInputChannelEnable.vi"("error in (no error)"=w344, "enable"=w347, "channel"=w346, "devidx"=w342) -> ("error out"=w345:errorcluster)  [unwired: 6 in, 1 out]
              }
              frame "SetInpChanOffset" {
                n162 = Unbundle By Name(w350) -> ("Offset"=w348:i32)
                n163 = call "MH_SetInputChannelOffset.vi"("error in (no error)"=w351, "Offset"=w348, "channel"=w353, "devidx"=w349) -> ("error out"=w352:errorcluster)  [unwired: 6 in, 1 out]
              }
              frame "SetInpChanDeadTime" {
                w356 = 32  # FEATURE_PROG_TD
                n164 = And(x=w355, y=w356) -> (x .and. y?=w357:i32)
                n165 = Not Equal To 0?(x=w357) -> (x != 0?=w354:bool)
                n166 = case shown="False" w354 {
                  tunnel: [w363 w372] -> w362
                  tunnel: w361 -> [w363 w371]
                  tunnel: w360 -> [_ w370]
                  tunnel: w359 -> [_ w369]
                  tunnel: w358 -> [_ w367]
                  frame False {
                  }
                  frame True {
                    n167 = Unbundle By Name(w370) -> ("UseDeadTime"=w366:bool, "DeadTime"=w368:i32)
                    n168 = Boolean To (0,1)(Boolean=w366) -> (0, 1=w365:i16)
                    n169 = To Long Integer(number=w365) -> (32bit integer=w364:i32)
                    n170 = call "MH_SetInputDeadTime.vi"("channel"=w367, "error in (no error)"=w371, "deadtime"=w368, "on"=w364, "devidx"=w369) -> ("error out"=w372:errorcluster)  [unwired: 5 in, 1 out]
                  }
                }
              }
              frame "SetInpChanTrg" {
                n171 = Unbundle By Name(w377) -> ("Level"=w373:i32, "Edge"=w375:i32)
                n172 = call "MH_SetInputEdgeTrg.vi"("channel"=w374, "error in (no error)"=w378, "edge"=w375, "level"=w373, "devidx"=w376) -> ("error out"=w379:errorcluster)  [unwired: 5 in, 1 out]
              }
            }
          }
        }
      }
      frame "SetSyncDivider" {
        n173 = Unbundle By Name(w387) -> ("DevIdx"=w386:i32, "SyncDivider"=w382:i32)
        n174 = Power Of 2(x=w382) -> (2^x=w381:dbl)
        n175 = To Long Integer(number=w381) -> (32bit integer=w380:i32)
        n176 = call "MH_SetSyncDiv.vi"("SyncDivider"=w380, "devidx"=w386) -> ("error out"=w384:errorcluster)  [unwired: 8 in, 1 out]
        n177 = flat-sequence {
          tunnel: w384 -> [w388]
          tunnel: [w388] -> w383
          frame #0 {
            n178 = Wait (ms)(milliseconds to wait=u32 100) -> ()  [unwired: 1 out]
          }
        }
      }
      frame "SetSyncTrg" {
        n179 = Unbundle By Name(w395) -> ("DevIdx"=w392:i32, "SyncLevel"=w390:i32, "SyncEdge"=w391:i32)
        n180 = call "MH_SetSyncEdgeTrg.vi"("edge"=w391, "level"=w390, "devidx"=w392) -> ("error out"=w393:errorcluster)  [unwired: 7 in, 1 out]
      }
      frame "SetSyncDeadTime" {
        w398 = 32  # FEATURE_PROG_TD
        n181 = Unbundle By Name(w407) -> ("DevIdx"=w404:i32, "UseDeadTime"=w402:bool, "SyncDeadTime"=w403:i32, "Init Info.features"=w397:i32)
        n182 = Boolean To (0,1)(Boolean=w402) -> (0, 1=w401:i16)
        n183 = And(x=w397, y=w398) -> (x .and. y?=w399:i32)
        n184 = To Long Integer(number=w401) -> (32bit integer=w400:i32)
        n185 = Not Equal To 0?(x=w399) -> (x != 0?=w396:bool)
        n186 = case shown="False" w396 {
          tunnel: [_ w411] -> w405
          tunnel: w404 -> [_ w410]
          tunnel: w403 -> [_ w409]
          tunnel: w400 -> [_ w408]
          frame False {
          }
          frame True {
            n187 = call "MH_SetSyncDeadTime.vi"("deadtime"=w409, "on"=w408, "devidx"=w410) -> ("error out"=w411:errorcluster)  [unwired: 7 in, 1 out]
          }
        }
      }
      frame "SetSyncOffset" {
        n188 = Unbundle By Name(w416) -> ("DevIdx"=w414:i32, "SyncOffset"=w413:i32)
        n189 = call "MH_SetSyncChannelOffset.vi"("Offset"=w413, "devidx"=w414) -> ("error out"=w415:errorcluster)  [unwired: 8 in, 1 out]
      }
      frame "SetBinning" {
        # "When binning is changed the new resolution is querried"
        n190 = Unbundle By Name(w423) -> ("DevIdx"=w421:i32, "Binning"=w420:i32)
        n191 = call "MH_SetBinning.vi"("Binning"=w420, "devidx"=w421) -> ("error out"=w422:errorcluster)  [unwired: 8 in, 1 out]
        n192 = Build Array (concatenate)(MH_UIThread_Cmds."GetResolution", w418) -> (w419:T8[])
      }
      frame "SetHistoOffset" {
        n193 = Unbundle By Name(w428) -> ("DevIdx"=w425:i32, "HistoOffset"=w424:i32)
        n194 = call "MH_SetOffset.vi"("Offset"=w424, "devidx"=w425) -> ("error out"=w426:errorcluster)  [unwired: 8 in, 1 out]
      }
      frame "SetHistoLen" {
        n195 = Unbundle By Name(w431) -> ("DevIdx"=w433:i32, "HistoLen"=w432:i32)
        n196 = call "MH_SetHistoLen.vi"("lencode"=w432, "devidx"=w433) -> ("error out"=w434:errorcluster, "actuallen"=w429:i32)  [unwired: 7 in, 1 out]
        n197 = Bundle By Name(cluster=w431, "HistoLength"=w429) -> (w430:T4)
      }
      frame "SetStopOvl" {
        n198 = Unbundle By Name(w441) -> ("DevIdx"=w438:i32, "StopOvl."=w437:bool, "OvlLevel"=w436:u32)
        n199 = call "MH_SetStopOverflow.vi"("stopcount"=w436, "StopOnOverflow"=w437, "devidx"=w438) -> ("error out"=w439:errorcluster)  [unwired: 7 in, 1 out]
      }
      frame "GetAllRates" {
        # "An alternative to GetRates"
        n200 = Unbundle By Name(w450) -> ("DevIdx"=w447:i32, "Init Info.nchannels"=w442:i32)
        n201 = call "MH_AllocateCntRateBuffer.vi"("NumChan"=w442) -> ("Buffer"=w443:i32[])  [unwired: 10 in]
        n202 = call "MH_GetAllCountRates.vi"("cntrates_buf"=w443, "devidx"=w447) -> ("error out"=w444:errorcluster, "cntrates"=→"CountRates":i32[], "syncrate"=w446:i32)  [unwired: 6 in, 1 out]
        n203 = Format Into String(format string="Sync Rate: %d cps\n", w446) -> (resulting string=→"SyncRate":string)  [unwired: 2 in, 1 out]
      }
      frame "GetRates" {
        # "An alternative to GetAllRates"
        n204 = Unbundle By Name(w461) -> ("Init Info.nchannels"=w456:i32, "Channels"=w458:T3[], "DevIdx"=w457:i32)
        n205 = call "MH_GetSyncRate.vi"("devidx"=w457) -> ("error out"=w454:errorcluster, "syncrate"=w453:i32)  [unwired: 8 in, 1 out]
        n206 = Format Into String(format string="Sync Rate: %d cps\n", w453) -> (resulting string=w455:string)  [unwired: 2 in, 1 out]
        n207 = for {
          N: w456 -> [_]
          tunnel: w457 -> [w468]
          tunnel: [w465] -> w452 mode=indexing
          shift-right: [w467] -> w460
          shift-left: w454 -> [w469]
          tunnel: w458 -> [w464] mode=indexing
          i -> [w466]
          n208 = Unbundle By Name(w464) -> ("Enable"=w463:bool)
          n209 = case shown="True" w463 {
            tunnel: w469 -> [w470 w475]
            tunnel: w468 -> [_ w474]
            tunnel: [w470 w473] -> w467
            tunnel: w466 -> [_ w472]
            tunnel: [_ w471] -> w465
            frame False {
            }
            frame True {
              n210 = call "MH_GetCountRate.vi"("error in (no error)"=w475, "Channel"=w472, "devidx"=w474) -> ("error out"=w473:errorcluster, "rate"=w471:i32)  [unwired: 6 in, 1 out]
            }
          }
        }
        n211 = local write "SyncRate"(w455) -> ()
        n212 = local write "CountRates"(w452) -> ()
      }
      frame "StartMeas" {
        n213 = Unbundle By Name(w483) -> ("AcqTime"=w479:i32, "DevIdx"=w480:i32)
        n214 = call "MH_ClearHistMem.vi"("devidx"=w480) -> ("error out"=w481:errorcluster)  [unwired: 9 in, 1 out]
        n215 = call "MH_StartMeas.vi"("error in (no error)"=w481, "tacq"=w479, "devidx"=w480) -> ("error out"=w482:errorcluster)  [unwired: 7 in, 1 out]
        n216 = Build Array (concatenate)(w478, MH_UIThread_Cmds."GetAllHistos") -> (w477:T8[])
      }
      frame "StopMeas" {
        n217 = Unbundle By Name(w489) -> ("Run cont."=w484:bool, "DevIdx"=w490:i32)
        n218 = call "MH_StopMeas.vi"("devidx"=w490) -> ("error out"=w491:errorcluster)  [unwired: 9 in, 1 out]
        n219 = case shown="False" w484 {
          tunnel: w489 -> [w495 w497]
          tunnel: [w494 w497] -> w488
          tunnel: [w492 w496] -> w487
          frame False {
            w492 = T8[] [enum."GetAllHistos"] items=["Idle", "Init", "SetInpChan", "SetSyncDivider", "SetSyncTrg", "SetSyncOffset", "SetSyncDeadTime", "SetBinning", "SetHistoOffset", "SetHistoLen", "SetStopOvl", "SetBitShift", "SetHistoAcqTime", "GetRates", "GetAllRates", "StartMeas", "StopMeas", "AbortMeas", "GetResolution", "GetHistos", "GetAllHistos", "ReadFiFo", "WriteStatus", "Resize", "EnableControls", "DisableControls", "Error", "Exit"]
            w493 = FALSE ("StartMeas")
            n220 = Bundle By Name(cluster=w495, "StartMeas"=w493) -> (w494:T4)
            n221 = local write "Start"(w493) -> ()
          }
          frame True {
            w496 = T8[] [enum."GetAllHistos", enum."StartMeas"] items=["Idle", "Init", "SetInpChan", "SetSyncDivider", "SetSyncTrg", "SetSyncOffset", "SetSyncDeadTime", "SetBinning", "SetHistoOffset", "SetHistoLen", "SetStopOvl", "SetBitShift", "SetHistoAcqTime", "GetRates", "GetAllRates", "StartMeas", "StopMeas", "AbortMeas", "GetResolution", "GetHistos", "GetAllHistos", "ReadFiFo", "WriteStatus", "Resize", "EnableControls", "DisableControls", "Error", "Exit"]
          }
        }
        n222 = Build Array (concatenate)(w486, w487) -> (w485:T8[])
      }
      frame "AbortMeas" {
        w501 = T8[] [enum."GetAllHistos"] items=["Idle", "Init", "SetInpChan", "SetSyncDivider", "SetSyncTrg", "SetSyncOffset", "SetSyncDeadTime", "SetBinning", "SetHistoOffset", "SetHistoLen", "SetStopOvl", "SetBitShift", "SetHistoAcqTime", "GetRates", "GetAllRates", "StartMeas", "StopMeas", "AbortMeas", "GetResolution", "GetHistos", "GetAllHistos", "ReadFiFo", "WriteStatus", "Resize", "EnableControls", "DisableControls", "Error", "Exit"]
        w498 = FALSE ("StartMeas")
        n223 = Unbundle By Name(w503) -> ("DevIdx"=w504:i32)
        n224 = call "MH_StopMeas.vi"("devidx"=w504) -> ("error out"=w505:errorcluster)  [unwired: 9 in, 1 out]
        n225 = Bundle By Name(cluster=w503, "StartMeas"=w498) -> (w502:T4)
        n226 = local write "Start"(w498) -> ()
        n227 = Build Array (concatenate)(w500, w501) -> (w499:T8[])
      }
      frame "GetResolution" {
        # "Resolution in ns"
        # "Gets resolution in ps"
        # "Resolution is saved in UIThread Data cluster in ns"
        n228 = Unbundle By Name(w510) -> ("DevIdx"=w512:i32)
        n229 = call "MH_GetResolution.vi"("devidx"=w512) -> ("error out"=w511:errorcluster, "resolution"=w508:dbl)  [unwired: 8 in, 1 out]
        n230 = Divide(x=w508, y=1000.0) -> (x/y=w506:dbl)
        n231 = Bundle By Name(cluster=w510, "Resolution"=w506) -> (w509:T4)
      }
      frame "GetAllHistos" {
        w526 = 1  # FLAG_OVERFLOW
        # "Provides a buffer (U32-array of length 'HistoLength' x nchannels) for all histograms."
        # "An alternative to GetHistos"
        n232 = Unbundle By Name(w537) -> ("Resolution"=w536:dbl, "DevIdx"=w516:i32, "HistoLength"=w519:i32, "Init Info.nchannels"=w520:i32)
        n233 = call "MH_AllocateAllHistoBuffer.vi"("NumChan"=w520, "HistoLength"=w519) -> ("Buffer"=w517:u32[])  [unwired: 9 in]
        n234 = call "MH_GetAllHistograms.vi"("Chcount"=w517, "devidx"=w516) -> ("error out"=w514:errorcluster, "Histograms"=w515:u32[])  [unwired: 7 in, 1 out]
        n235 = Reshape Array(w515, w520, w519) -> (w518:u32[][])
        n236 = for {
          tunnel: [w539] -> w528 mode=indexing
          shift-right: [w541] -> w522
          shift-left: "Total Counts:\t\t" -> [w540]
          tunnel: w518 -> [w539] mode=indexing
          i -> [w545]
          n237 = Add Array Elements(numeric array=w539) -> (sum=w542:u32)
          n238 = Increment(x=w545) -> (x+1=w543:i32)
          n239 = Format Into String(format string="Ch.%2d: %d cnts.\t\t", initial string=w540, w543, w542) -> (resulting string=w541:string)  [unwired: 1 in, 1 out]
        }
        n240 = call "CalcRate.vi"("Refresh(ms)"=u32 500) -> ("Rate / Hz"=w534:dbl)  [unwired: 8 in, 2 out]
        n241 = Format Into String(format string="Readout Rate: %.1f Hz\\t\\t", w534) -> (resulting string=w532:string)  [unwired: 2 in, 1 out]
        n242 = Concatenate Strings(w532, w522) -> (w531:string)
        n243 = Bundle(0.0, "Resolution"=w536, "Histograms"=w528) -> (→"HistoGraph":T13)  [unwired: 1 in]
        n244 = local write "Status"(w531) -> ()
        n245 = call "MH_GetFlags.vi"("error in (no error)"=w514) -> ("error out"=w535:errorcluster, "flags"=w525:i32)  [unwired: 8 in, 1 out]
        n246 = And(x=w526, y=w525) -> (x .and. y?=w527:i32)
        n247 = Not Equal To 0?(x=w527) -> (x != 0?=→"OverFlow":bool)
      }
      frame "GetHistos" {
        w555 = 1  # FLAG_OVERFLOW
        # "Provides a buffer (U32-array of length 'HistoLength') for histograms."
        # "An alternative to GetAllHistos"
        n248 = Unbundle By Name(w569) -> ("Resolution"=w566:dbl, "Init Info.nchannels"=w548:i32, "Channels"=w549:T3[], "DevIdx"=w568:i32, "HistoLength"=w567:i32)
        n249 = call "MH_AllocateHistoBuffer.vi"("HistoLength"=w567) -> ("Buffer"=w560:u32[])  [unwired: 10 in]
        n250 = for {
          N: w548 -> [_]
          tunnel: w568 -> [w583]
          tunnel: [w571] -> w558 mode=indexing
          tunnel: w560 -> [w581]
          shift-right: [w582] -> w557
          shift-left: errorcluster {"status"=FALSE, "code"=0, "source"=""} ("error IO") -> [w575]
          shift-right: [w576] -> w551
          shift-left: "Total Counts:\t\t" -> [w574]
          tunnel: w549 -> [w573] mode=indexing
          i -> [w580]
          n251 = Unbundle By Name(w573) -> ("Enable"=w572:bool)
          n252 = case shown="True" w572 {
            tunnel: w583 -> [_ w591]
            tunnel: [w584 w590] -> w582
            tunnel: w581 -> [w585 w589]
            tunnel: [w585 w588] -> w571
            tunnel: w580 -> [_ w587]
            tunnel: w575 -> [w584 w586]
            frame False {
            }
            frame True {
              n253 = call "MH_GetHistogram.vi"("Chcount"=w589, "error in (no error)"=w586, "channel"=w587, "devidx"=w591) -> ("error out"=w590:errorcluster, "Histogram"=w588:u32[])  [unwired: 5 in, 1 out]
            }
          }
          n254 = Add Array Elements(numeric array=w571) -> (sum=w577:u32)
          n255 = Increment(x=w580) -> (x+1=w578:i32)
          n256 = Format Into String(format string="Ch.%2d: %d cnts.\t\t", initial string=w574, w578, w577) -> (resulting string=w576:string)  [unwired: 1 in, 1 out]
        }
        n257 = call "CalcRate.vi"("Refresh(ms)"=u32 500) -> ("Rate / Hz"=w564:dbl)  [unwired: 8 in, 2 out]
        n258 = Format Into String(format string="Readout Rate: %.1f Hz\\t\\t", w564) -> (resulting string=w562:string)  [unwired: 2 in, 1 out]
        n259 = Concatenate Strings(w562, w551) -> (w561:string)
        n260 = Bundle(0.0, "Resolution"=w566, "Histogram"=w558) -> (w546:T2)  [unwired: 1 in]
        n261 = local write "HistoGraph"(w546) -> ()
        n262 = local write "Status"(w561) -> ()
        n263 = call "MH_GetFlags.vi"("error in (no error)"=w557) -> ("error out"=w565:errorcluster, "flags"=w554:i32)  [unwired: 8 in, 1 out]
        n264 = And(x=w555, y=w554) -> (x .and. y?=w556:i32)
        n265 = Not Equal To 0?(x=w556) -> (x != 0?=w547:bool)
        n266 = local write "OverFlow"(w547) -> ()
      }
      frame "WriteStatus" {
        n267 = Unbundle By Name(w593) -> ("Status"=→"Status":string)
      }
      frame "Resize" {
        n268 = property on="Pane 3" class="Pane"() -> ("Width"=w600:u32)  [unwired: 2 in, 2 out]
        n269 = Subtract(x=w600, y=i16 100 ("b")) -> (x-y=w606:u32)
        n270 = Unbundle By Name(w595) -> ("Init Info.nchannels"=w603:i32)
        n271 = Quotient & Remainder(x=w606, y=i16 99 ("m")) -> (floor(x/y)=w605:u32)  [unwired: 1 out]
        n272 = In Range and Coerce(upper limit=w603, x=w605, lower limit=4) -> (coerced(x)=w604:u32)  [unwired: 1 out]
        n273 = Equal?(x=w603, y=w604) -> (x = y?=w602:bool)
        n274 = Not(x=w602) -> (.not. x?=w601:bool)
        n275 = property on="Channels" class="Arr (strict)"("HorizScroll"=w601, "Number of Columns"=w604, "Index Values"=u32[] [0]) -> ()  [unwired: 2 in, 2 out]
      }
      frame "EnableControls" {
        n276 = property class="VI"() -> ("Panel"=w611:refnum<vi>)  [unwired: 2 in, 2 out]
        n277 = property class="Pnl"(reference=w611) -> ("Controls[]"=w610:refnum<vi>[])  [unwired: 1 in, 2 out]
        n278 = property class="Pnl"(reference=w611) -> ("Decos[]"=w612:refnum<vi>[])  [unwired: 1 in, 2 out]
        n279 = for {
          tunnel: w612 -> [w616] mode=indexing
          tunnel: TRUE -> [w615]
          n280 = property class="Decor"(reference=w616, "Visible"=w615) -> ()  [unwired: 1 in, 2 out]
        }
        n281 = for {
          tunnel: w610 -> [w619] mode=indexing
          tunnel: T9."Enabled" ("Disabled") -> [w618]
          tunnel: [w617] -> _
          n282 = property class="Ctl"(reference=w619, "DisabledEnum"=w618) -> (error out=w617:errorcluster)  [unwired: 1 in, 1 out]
        }
      }
      frame "DisableControls" {
        n283 = property class="VI"() -> ("Panel"=w623:refnum<vi>)  [unwired: 2 in, 2 out]
        n284 = property class="Pnl"(reference=w623) -> ("Controls[]"=w622:refnum<vi>[])  [unwired: 1 in, 2 out]
        n285 = property class="Pnl"(reference=w623) -> ("Decos[]"=w624:refnum<vi>[])  [unwired: 1 in, 2 out]
        n286 = for {
          tunnel: w624 -> [w628] mode=indexing
          tunnel: FALSE -> [w627]
          n287 = property class="Decor"(reference=w628, "Visible"=w627) -> ()  [unwired: 1 in, 2 out]
        }
        n288 = for {
          tunnel: w622 -> [w631] mode=indexing
          tunnel: T9."Disabled and Grayed Out" ("Disabled") -> [w630]
          tunnel: [w629] -> _
          n289 = property class="Ctl"(reference=w631, "DisabledEnum"=w630) -> (error out=w629:errorcluster)  [unwired: 1 in, 1 out]
        }
      }
      frame "Error" {
        w632 = T8[] [enum."Exit"] items=["Idle", "Init", "SetInpChan", "SetSyncDivider", "SetSyncTrg", "SetSyncOffset", "SetSyncDeadTime", "SetBinning", "SetHistoOffset", "SetHistoLen", "SetStopOvl", "SetBitShift", "SetHistoAcqTime", "GetRates", "GetAllRates", "StartMeas", "StopMeas", "AbortMeas", "GetResolution", "GetHistos", "GetAllHistos", "ReadFiFo", "WriteStatus", "Resize", "EnableControls", "DisableControls", "Error", "Exit"]
        w635 = T14 1 items=["no dialog", "OK message", "continue or stop message", "OK message + warnings", "continue/stop + warnings"] ("type of dialog (OK msg:1)")
        # "Error case: If an error occures the user is informed and the programm terminates. Add your own code to handle error events (e.g. exception lists, etc.)"
        n290 = call <vilib>:"Simple Error Handler.vi"("type of dialog (OK msg:1)"=w635, "error in (no error)"=w634) -> ()  [unwired: 3 in, 5 out]
      }
      frame "Exit" {
        n291 = Unbundle By Name(w639) -> ("DevIdx"=w638:i32)
        n292 = call "MH_CloseDevice.vi"("devidx"=w638) -> ("error out"=w637:errorcluster)  [unwired: 9 in, 1 out]
      }
    }
    n293 = call "MH_EnQError.vi"("error in (no error)"=w8, "Cmds_in"=w6) -> ("error out"=w7:errorcluster, "Cmds_out"=w5:T8[])  [unwired: 8 in]
  }
